vi "backward.vi"(0 "a1":dbl, 1 "a2":dbl, 2 "T":dbl, 5 "Vi(n-1)":dbl, 7 "Vo(n-1)":dbl, 9 "b1":dbl, 12 "Vo(n-2)":dbl, 13 "Vo(n-3)":dbl, 14 "a0":dbl) -> (4 "Vo (salida)":dbl)   [LabVIEW 2011]
panel:
  # "Vo =                   Vi*b1\n             --------------------------\n             s^3  + a2*s^2 + a1*s + a0"
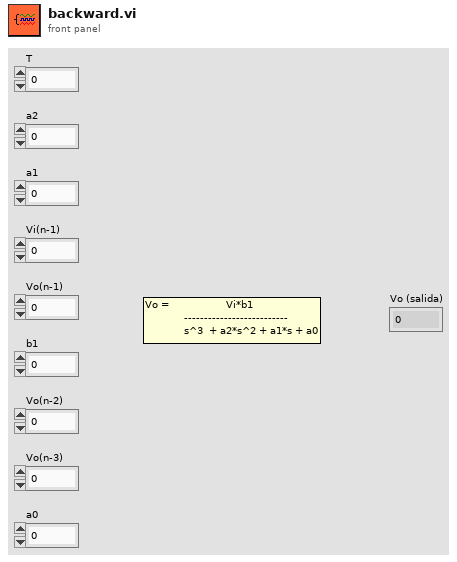
[diagram p1: front panel]
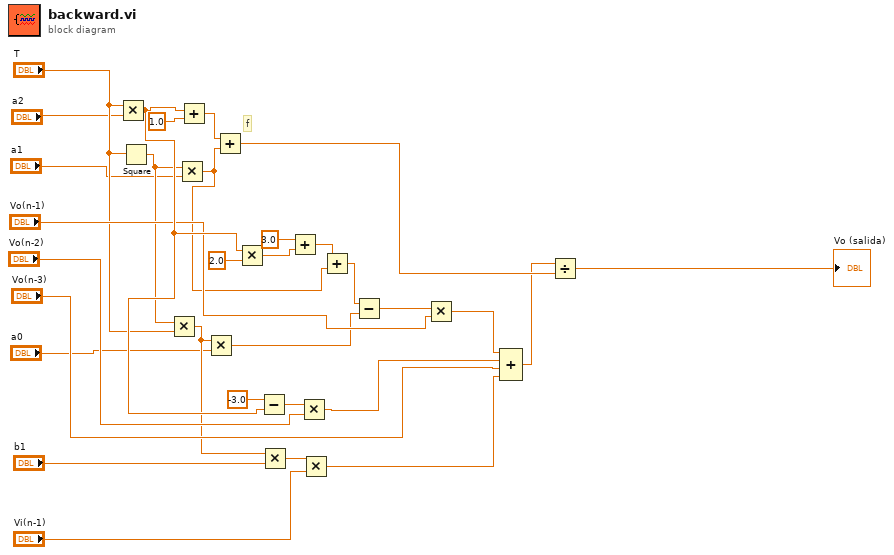
[diagram p0: block diagram]
diagram:
  # "f"
  n1 = Multiply(x="T", y="a2") -> (x*y=w30:dbl)
  n2 = Square(x="T") -> (x^2=w9:dbl)
  n3 = Multiply(x=w9, y="T") -> (x*y=w15:dbl)
  n4 = Multiply(x=w9, y="a1") -> (x*y=w8:dbl)
  n5 = Add(x=w30, y=1.0 ("x")) -> (x+y=w4:dbl)
  n6 = Multiply(x=w15, y="a0") -> (x*y=w13:dbl)
  n7 = Add(x=w4, y=w8) -> (x+y=w28:dbl)
  n8 = Multiply(x=w30, y=2.0) -> (x*y=w6:dbl)
  n9 = Subtract(x=-3.0, y=w30) -> (x-y=w19:dbl)
  n10 = Multiply(x=w15, y="b1") -> (x*y=w24:dbl)
  n11 = Add(x=3.0, y=w6) -> (x+y=w7:dbl)
  n12 = Multiply(x=w19, y="Vo(n-2)") -> (x*y=w22:dbl)
  n13 = Multiply(x=w24, y="Vi(n-1)") -> (x*y=w25:dbl)
  n14 = Add(x=w7, y=w8) -> (x+y=w12:dbl)
  n15 = Subtract(x=w12, y=w13) -> (x-y=w17:dbl)
  n16 = Multiply(x=w17, y="Vo(n-1)") -> (x*y=w21:dbl)
  n17 = Compound Arithmetic op=ADD(w21, w22, "Vo(n-3)", w25) -> (w27:dbl)
  n18 = Divide(x=w27, y=w28) -> (x/y=→"Vo (salida)":dbl)
